vi "_Find Row.vi"(8 "error in":errorcluster, 9 "Index":i32, 10 "SheetData":refnum<k24>) -> (0 "error out":errorcluster, 2 "Row":refnum<k24>)   [LabVIEW 2021, in "Open Xml.lvlib"]
uses:
  Open Xml.lvlib
  D:/git/Open-Xml-LabVIEW/DocumentFormat.OpenXml.dll
  DocumentFormat.OpenXml.dll
  D:/git/Open-Xml-LabVIEW/DocumentFormat.OpenXml.Framework.dll
  DocumentFormat.OpenXml.Framework.dll
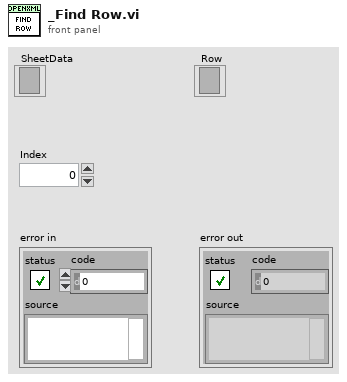
[diagram p1: front panel]
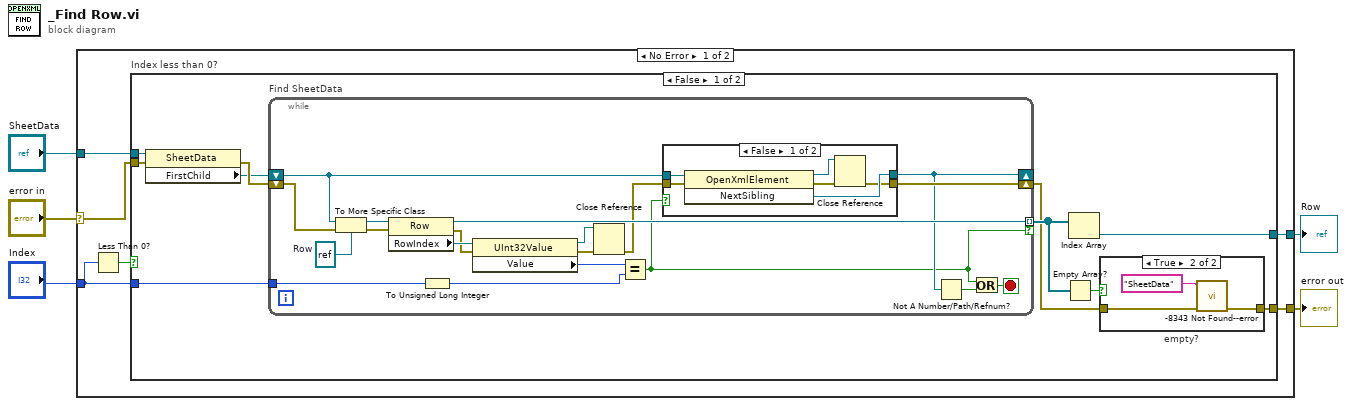
[diagram p0: block diagram]
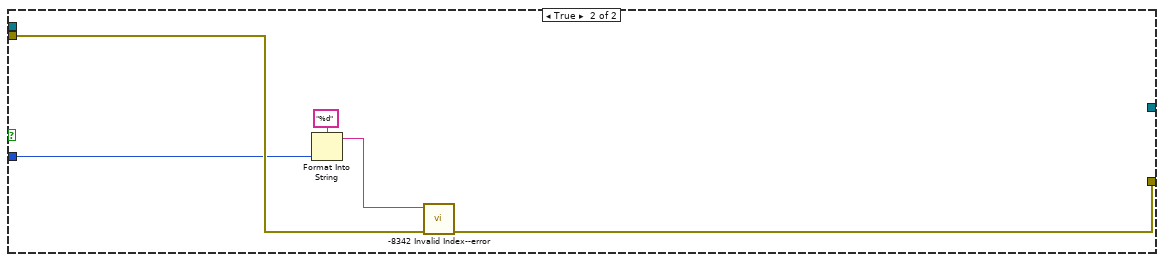
[diagram p4: hidden frame]
diagram:
  n1 = case shown="No Error" "error in" {
    selector: "error in" -> [w11 w58]
    tunnel: "SheetData" -> [w10 _]
    tunnel: [w9 _] -> w3
    tunnel: "Index" -> [w7 _]
    tunnel: [w6 w58] -> w1
    frame No Error {
      n2 = Less Than 0?(x=w7) -> (x < 0?=w8:bool)
      n3 = case "Index less than 0?" shown="False" w8 {
        tunnel: w11 -> [w19 w57]
        tunnel: w10 -> [w17 _]
        tunnel: w7 -> [w16 w55]
        tunnel: [w15 _] -> w9
        tunnel: [w12 w56] -> w6
        frame False {
          n4 = property class="SheetData"(reference=w17, error in=w19) -> (error out=w21:errorcluster, "FirstChild"=w20:refnum<k24>)  [unwired: 1 out]
          n5 = while "Find SheetData" {
            shift-right: [w32] -> w13
            shift-left: w21 -> [w44]
            shift-right: [w30] -> _
            shift-left: w20 -> [w31]
            tunnel: [w39] -> w18 mode=indexing if=w29
            tunnel: w16 -> [w34]
            stop <- w42 stop-if-true
            w41 = refnum<k24> refnum  # Row
            n6 = To More Specific Class(target class=w41, reference=w31, error in=w44) -> (specific class reference=w40:refnum<k24>, error out=w36:errorcluster)
            n7 = property class="Row"(reference=w40, error in=w36) -> (reference out=w39:refnum<k24>, error out=w37:errorcluster, "RowIndex"=w38:refnum<k24>)
            n8 = To Unsigned Long Integer(number=w34) -> (unsigned 32bit integer=w27:u32)
            n9 = property class="UInt32Value"(reference=w38, error in=w37) -> (reference out=w26:refnum<k24>, error out=w33:errorcluster, "Value"=w35:u32)
            n10 = Close Reference(reference=w26, error in (no error)=w33) -> (error out=w28:errorcluster)
            n11 = Equal?(x=w35, y=w27) -> (x = y?=w29:bool)
            n12 = case shown="False" w29 {
              tunnel: w28 -> [w50 w51]
              tunnel: [w46 w51] -> w32
              tunnel: [w47 w52] -> w30
              tunnel: w31 -> [w48 w52]
              frame False {
                n13 = invoke class="OpenXmlElement" method="NextSibling"(reference=w48, error in=w50) -> (reference out=w45:refnum<k24>, error out=w49:errorcluster, "NextSibling"=w47:refnum<k24>)  [unwired: 1 in]
                n14 = Close Reference(reference=w45, error in (no error)=w49) -> (error out=w46:errorcluster)
              }
              frame True {
              }
            }
            n15 = Not A Number/Path/Refnum?(number/path/refnum=w30) -> (NaN/Path/Refnum?=w43:bool)
            n16 = Or(x=w29, y=w43) -> (x .or. y?=w42:bool)
          }
          n17 = Empty Array?(array=w18) -> (empty?=w14:bool)
          n18 = Index Array(array=w18) -> (element=w15:refnum<k24>)  [unwired: 1 in]
          n19 = case "empty?" shown="True" w14 {
            tunnel: w13 -> [w22 w25]
            tunnel: [w22 w24] -> w12
            frame False {
            }
            frame True {
              n20 = call "-8343 Not Found--error.vi"("error in (no error)"=w25, "Item"="SheetData") -> ("error out"=w24:errorcluster)  [unwired: 9 in]
            }
          }
        }
        frame True {
          n21 = Format Into String(format string="%d", w55) -> (resulting string=w54:string)  [unwired: 2 in, 1 out]
          n22 = call "-8342 Invalid Index--error.vi"("error in"=w57, "Index"=w54) -> ("error out"=w56:errorcluster)  [unwired: 9 in]
        }
      }
    }
    frame Error {
    }
  }
  "error out" <- w1
  "Row" <- w3
